vi "Convert_Existing_TDMS.vi"(8 "This VI":refnum<vi>, 11 "TDMS DataFile Name":path) -> ()   [LabVIEW 2023]
uses:
  Settings.vi
panel:
  out "error out 2":errorcluster
  out "error out":errorcluster
  out "Save a copy of the Binary Data File":bool
  out "PointsPerRow":u64
  out "NumberOfRowstoSave":i16
  out "ApproxBytes":dbl
  out "Save File Path":path
  out "Save Channels Separatly":bool
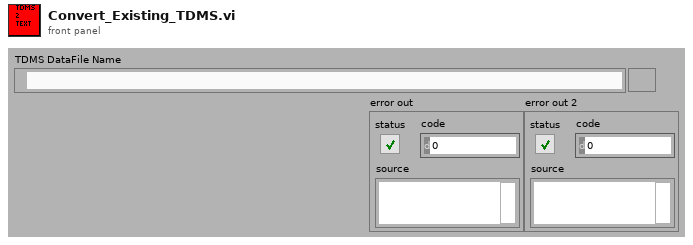
[diagram p1: front panel]
types:
  T1 = enum16{"open", "open or create", "create or replace", "create", "open (read-only)"}
  T2 = enum16{"open", "replace", "create", "open or create", "replace or create", "replace or create with confirmation"}
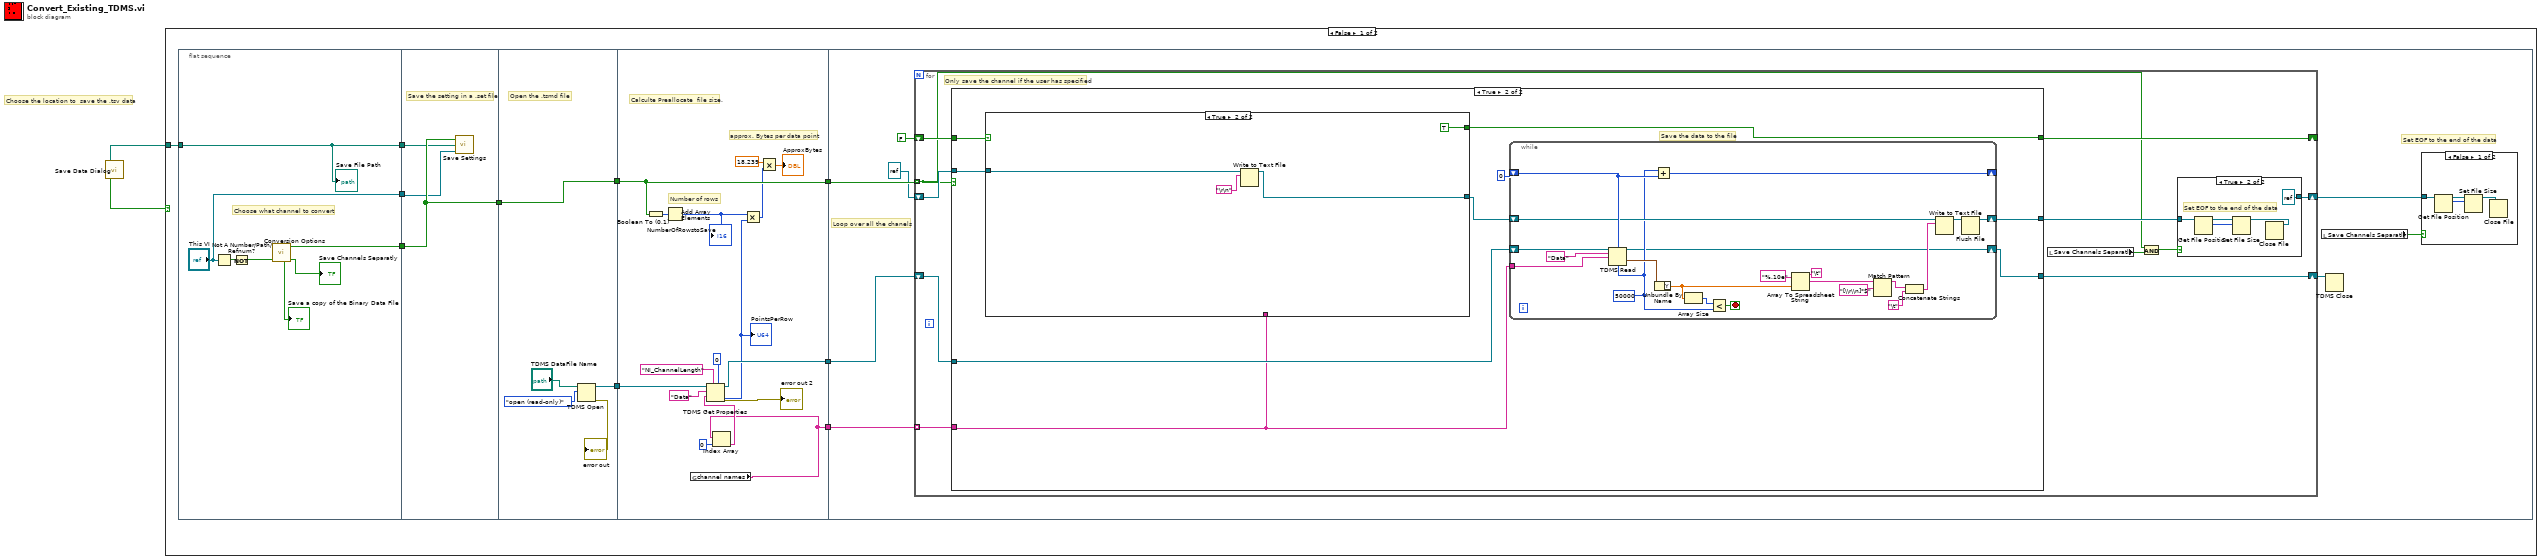
[diagram p0: block diagram]
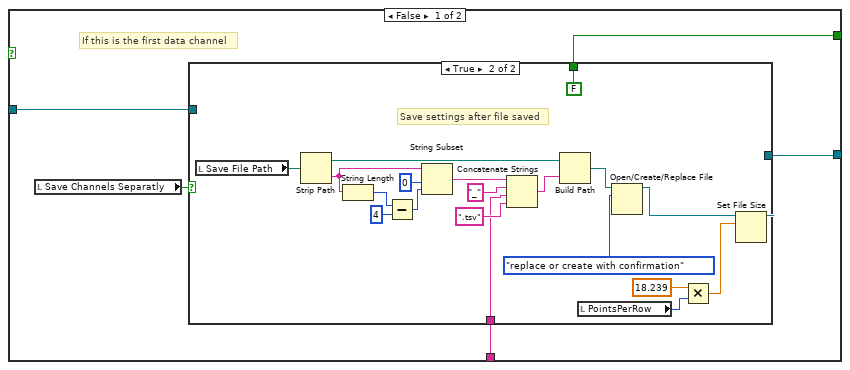
[diagram p5: hidden frame]
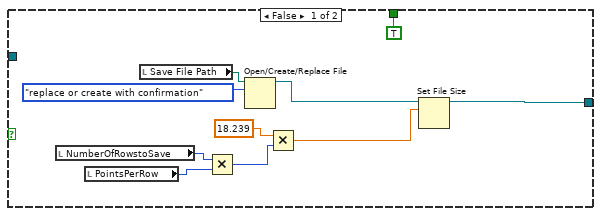
[diagram p6: hidden frame]
diagram:
  # "Choose the location to  save the .tsv data"
  n1 = call "Save Data Dialog.vi"() -> ("cancelled"=w2:bool, "selected path"=w1:path)  [unwired: 1 in]
  n2 = case shown="False" w2 {
    tunnel: w1 -> [w4 _]
    frame False {
      n3 = flat-sequence {
        tunnel: [w17] -> w7
        tunnel: ["This VI"] -> w6
        tunnel: w4 -> [w13]
        tunnel: [w13] -> w3
        tunnel: [w22] -> w8
        tunnel: w7 -> [w22]
        tunnel: w6 -> [w21]
        tunnel: w3 -> [w20]
        tunnel: [w25] -> w12
        tunnel: [w26] -> w9
        tunnel: w8 -> [w25]
        tunnel: w12 -> [w43]
        tunnel: [w43] -> w11
        tunnel: [w38] -> w10
        tunnel: w9 -> [w41]
        tunnel: [w29] -> w5
        tunnel: w11 -> [w51]
        tunnel: w10 -> [w49]
        tunnel: w5 -> [w44]
        frame #0 {
          # "Choose what channel to convert"
          n4 = Not A Number/Path/Refnum?(number/path/refnum="This VI") -> (NaN/Path/Refnum?=w19:bool)
          n5 = Not(x=w19) -> (.not. x?=w16:bool)
          n6 = call "Conversion Options.vi"("Save a copy of the Binary Data File"=w16) -> ("Save Each Channel as a Separate File indicator"=→"Save Channels Separatly":bool, "Array"=w17:bool[], "Save a copy of the Binary Data File"=→"Save a copy of the Binary Data File":bool)  [unwired: 8 in]
          "Save File Path" <- w13
        }
        frame #1 {
          # "Save the setting in a .set file"
          n7 = call "Save Settings.vi"("This VI"=w21, "Path"=w20, "Array"=w22) -> ()  [unwired: 1 in]
        }
        frame #2 {
          # "Open the .tsmd file"
          n8 = TDMS Open(10:T1."open (read-only)" ("operation (0:open)"), 11:"TDMS DataFile Name") -> (0:→"error out":errorcluster, 3:w26:refnum<k34>)  [unwired: 5 in]
        }
        frame #3 {
          # "approx. Bytes per data point"
          # "Number of rows"
          # "Calculte Preallocate  file size."
          n9 = Boolean To (0,1)(Boolean=w43) -> (0, 1=w42:i16[])
          n10 = Add Array Elements(numeric array=w42) -> (sum=w35:i16)
          "NumberOfRowstoSave" <- w35
          n11 = global read "Settings.vi" "channel names"() -> (w29:string[])
          n12 = Index Array(array=w29, index=0) -> (element=w30:string)
          n13 = TDMS Get Properties(5:u64 0, 7:"NI_ChannelLength" ("property name"), 9:w30, 10:"Data" ("group name in"), 11:w41) -> (0:→"error out 2":errorcluster, 3:w38:refnum<k34>, 4:w36:u64)  [unwired: 1 in, 3 out]
          "PointsPerRow" <- w36
          n14 = Multiply(x=w35, y=w36) -> (x*y=w34:u64)
          n15 = Multiply(x=18.239, y=w34) -> (x*y=→"ApproxBytes":dbl)
        }
        frame #4 {
          # "Loop over all the chanels"
          # "Set EOF to the end of the data"
          n16 = for {
            tunnel: w51 -> [w58] mode=indexing
            shift-right: [w65] -> _
            shift-left: FALSE -> [w66]
            tunnel: w44 -> [w64] mode=indexing
            shift-right: [w56] -> w47
            shift-left: refnum<file> refnum ("refnum out") -> [w63]
            shift-right: [w61] -> w48
            shift-left: w49 -> [w62]
            # "Only save the channel if the user has specified"
            n17 = case shown="True" w58 {
              tunnel: w64 -> [_ w76]
              tunnel: w66 -> [w75 w84]
              tunnel: [w75 w77] -> w65
              tunnel: [w74 w80] -> w60
              tunnel: w63 -> [w74 w83]
              tunnel: w62 -> [w73 w79]
              tunnel: [w73 w78] -> w61
              frame False {
              }
              frame True {
                # "Save the data to the file"
                n18 = case shown="True" w84 {
                  tunnel: w83 -> [w108 w144]
                  tunnel: [w110 w143] -> w81
                  tunnel: [w109 TRUE] -> w77
                  tunnel: w76 -> [w106 _]
                  frame False {
                    # "If this is the first data channel"
                    n19 = local read "Save Channels Separatly"() -> (w107:bool)
                    n20 = case shown="True" w107 {
                      tunnel: w108 -> [_ _]
                      tunnel: [w117 w122] -> w110
                      tunnel: [TRUE FALSE] -> w109
                      tunnel: w106 -> [_ w121]
                      frame False {
                        n21 = local read "NumberOfRowstoSave"() -> (w115:i16)
                        n22 = local read "PointsPerRow"() -> (w114:u64)
                        n23 = local read "Save File Path"() -> (w119:path)
                        n24 = Multiply(x=w115, y=w114) -> (x*y=w113:u64)
                        n25 = Open/Create/Replace File(file path (use dialog)=w119, operation (0:open)=T2."replace or create with confirmation") -> (refnum out=w118:refnum<file>)  [unwired: 4 in, 2 out]
                        n26 = Multiply(x=18.239, y=w113) -> (x*y=w111:dbl)
                        n27 = Set File Size(6:w111, 7:w118) -> (3:w117:refnum<file>)  [unwired: 1 in, 1 out]
                      }
                      frame True {
                        # "Save settings after file saved"
                        n28 = local read "Save File Path"() -> (w131:path)
                        n29 = Strip Path(path=w131) -> (stripped path=w132:path, name=w136:string)
                        n30 = String Length(string=w136) -> (length=w137:i32)
                        n31 = Subtract(x=w137, y=4) -> (x-y=w138:i32)
                        n32 = String Subset(string=w136, offset (0)=0, length (rest)=w138) -> (substring=w134:string)
                        n33 = Concatenate Strings(w134, "_" ("string"), w121, ".tsv") -> (w133:string)
                        n34 = Build Path(base path=w132, name or relative path=w133) -> (appended path=w126:path)
                        n35 = local read "PointsPerRow"() -> (w125:u64)
                        n36 = Open/Create/Replace File(file path (use dialog)=w126, operation (0:open)=T2."replace or create with confirmation") -> (refnum out=w127:refnum<file>)  [unwired: 4 in, 2 out]
                        n37 = Multiply(x=18.239, y=w125) -> (x*y=w123:dbl)
                        n38 = Set File Size(6:w123, 7:w127) -> (3:w122:refnum<file>)  [unwired: 1 in, 1 out]
                      }
                    }
                  }
                  frame True {
                    n39 = Write to Text File(file (use dialog)=w144, text="\r\n") -> (refnum out=w143:refnum<file>)  [unwired: 2 in, 2 out]
                  }
                }
                n40 = while {
                  tunnel: w76 -> [w105]
                  shift-right: [w87] -> w78
                  shift-left: w79 -> [w104]
                  shift-right: [w101] -> w80
                  shift-left: w81 -> [w91]
                  shift-right: [w103] -> _
                  shift-left: i64 0 ("offset (0)") -> [w102]
                  stop <- w98 stop-if-true
                  w88 = i64 50000 ("count (-1: all)")
                  n41 = TDMS Read(0:w104, 1:w102, 2:w88, 5:"Data" ("group name in"), 7:w105) -> (4:w87:refnum<k34>, 10:w99:waveform(dbl))  [unwired: 3 in, 4 out]
                  n42 = Add(x=w88, y=w102) -> (x+y=w103:i64)
                  n43 = Unbundle By Name(w99) -> ("Y"=w86:dbl[])
                  n44 = Array Size(array=w86) -> (size(s)=w97:i32)
                  n45 = Less?(x=w97, y=w88) -> (x < y?=w98:bool)
                  n46 = Array To Spreadsheet String(delimiter (Tab)="\t", array=w86, 3:"%.10e") -> (spreadsheet string=w93:string)
                  n47 = Match Pattern(string=w93, regular expression="[\\r\\n]*$") -> (before substring=w94:string)  [unwired: 1 in, 3 out]
                  n48 = Concatenate Strings(w94, "\t") -> (w90:string)
                  n49 = Write to Text File(file (use dialog)=w91, text=w90) -> (refnum out=w89:refnum<file>)  [unwired: 2 in, 2 out]
                  n50 = Flush File(refnum=w89) -> (refnum out=w101:refnum<file>)  [unwired: 1 in, 1 out]
                }
              }
            }
            n51 = local read "Save Channels Separatly"() -> (w59:bool)
            n52 = And(x=w58, y=w59) -> (x .and. y?=w57:bool)
            n53 = case shown="True" w57 {
              tunnel: w60 -> [w67 w69]
              tunnel: [w67 refnum<file> refnum ("refnum out")] -> w56
              frame False {
              }
              frame True {
                # "Set EOF to the end of the data"
                n54 = Get File Position(7:w69) -> (2:w71:i64, 3:w70:refnum<file>)  [unwired: 1 in, 1 out]
                n55 = Set File Size(6:w71, 7:w70) -> (3:w72:refnum<file>)  [unwired: 1 in, 1 out]
                n56 = Close File(refnum=w72) -> ()  [unwired: 1 in, 2 out]
              }
            }
          }
          n57 = local read "Save Channels Separatly"() -> (w45:bool)
          n58 = TDMS Close(11:w48) -> ()  [unwired: 1 in, 2 out]
          n59 = case shown="False" w45 {
            tunnel: w47 -> [w55 _]
            frame False {
              n60 = Get File Position(7:w55) -> (2:w53:i64, 3:w54:refnum<file>)  [unwired: 1 in, 1 out]
              n61 = Set File Size(6:w53, 7:w54) -> (3:w52:refnum<file>)  [unwired: 1 in, 1 out]
              n62 = Close File(refnum=w52) -> ()  [unwired: 1 in, 2 out]
            }
            frame True {
            }
          }
        }
      }
    }
    frame True {
    }
  }
